vi "VHMI-recieveConnectionInfo.vi"(8 "error in (no error)":errorcluster, 10 "connection status":T1, 11 "VG-VNA_GUI in":refnum<class "VG-VNA_GUI.lvclass">) -> (0 "error out":errorcluster, 3 "VG-VNA_GUI out":refnum<class "VG-VNA_GUI.lvclass">)   [LabVIEW 2020, in "VG-VNA_GUI.lvlib" / "VG-VNA_GUI.lvclass"]
uses:
  VG-VNA_GUI.lvclass
  hardware_manager/VHM-VNA_Hardware_Manager/VHM-VNA_Hardware_Manager/VHM-connection_status.ctl
  hardware_manager/VHM-VNA_Hardware_Manager/VHM-VNA_Hardware_Manager/VHM-VNA_Hardware_Manager.lvclass
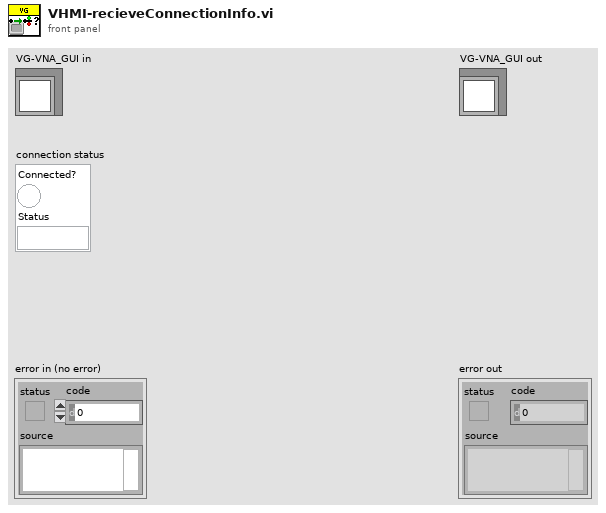
[diagram p1: front panel]
types:
  T1 = typedef "VHM-VNA_Hardware_Manager.lvlib/VHM-VNA_Hardware_Manager.lvclass/VHM-connection_status.ctl" = cluster{"Connected?":bool, "Status":string}
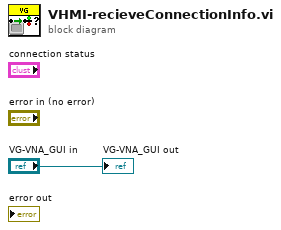
[diagram p0: block diagram]
diagram:
  "VG-VNA_GUI out" <- "VG-VNA_GUI in"
